vi "Opg5.vi"() -> ()   [LabVIEW 2022 SP3]
uses:
  <vilib>/numeric/Random Number (Range) U64.vi
  <vilib>/numeric/sub_Random U32.vi
panel:
  out "floor(x/y)":i32
  out "Array 2":i32[](array[numeric])
  out "Array":i32[](array[numeric])
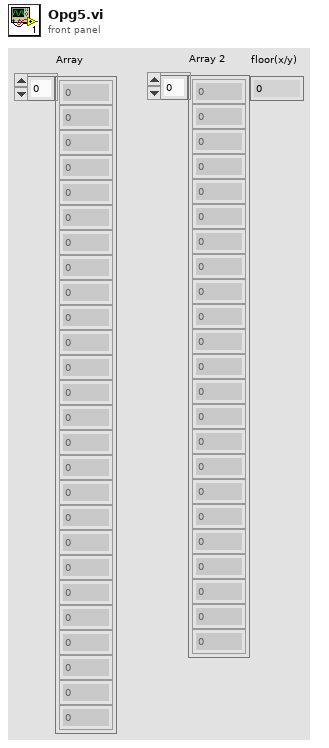
[diagram p1: front panel]
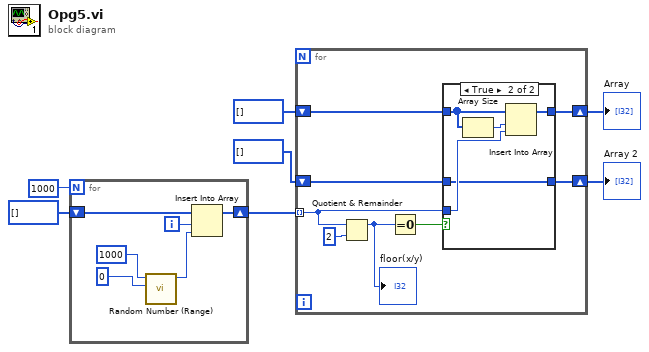
[diagram p0: block diagram]
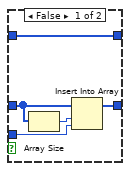
[diagram p2: hidden frame]
diagram:
  n1 = for {
    N: 1000 -> [_]
    shift-right: [w8] -> w5
    shift-left: i32[] [] -> [w9]
    i -> [w13]
    n2 = call-poly <vilib>:"Random Number (Range).vi"("lower bound (0)"=u64 0, "upper bound (100)"=u64 1000) -> ("number"=w12:u64)  [unwired: 9 in]
    n3 = Insert Into Array(array=w9, index=w13, new element=w12) -> (w8:i32[])
  }
  n4 = for {
    tunnel: w5 -> [w16] mode=indexing
    shift-right: [w17] -> w1
    shift-left: i32[] [] -> [w18]
    shift-right: [w19] -> w2
    shift-left: i32[] [] -> [w20]
    n5 = Quotient & Remainder(x=w16, y=2) -> (x-y*floor(x/y)=w14:i32)  [unwired: 1 out]
    "floor(x/y)" <- w14
    n6 = Equal To 0?(x=w14) -> (x = 0?=w21:bool)
    n7 = case shown="True" w21 {
      tunnel: w16 -> [w24 w30]
      tunnel: w20 -> [w23 w29]
      tunnel: [w23 w28] -> w19
      tunnel: w18 -> [w25 w27]
      tunnel: [w22 w27] -> w17
      frame False {
        n8 = Array Size(array=w25) -> (size(s)=w26:i32)
        n9 = Insert Into Array(array=w25, index=w26, new element=w24) -> (w22:i32[])
      }
      frame True {
        n10 = Array Size(array=w29) -> (size(s)=w31:i32)
        n11 = Insert Into Array(array=w29, index=w31, new element=w30) -> (w28:i32[])
      }
    }
  }
  "Array" <- w2
  "Array 2" <- w1
